vi "Edit papers.vi"(8 "Error In":errorcluster, 11 "INI refnum in":T1) -> (0 "Error Out":errorcluster, 3 "INI refnum Out":T1)   [LabVIEW 2015]
uses:
  <vilib>/Utility/config.llb/Config Data RefNum.ctl
  Edit papers state.ctl
  <vilib>/Utility/miscctls.llb/LVMenuShortCut.ctl
  <vilib>/Utility/config.llb/NI_LVConfig.lvlib
panel:
  in  "Clear table":bool
  in  "Exit":bool
  in  "Discared changes":bool
  in  "Save":bool
  in  "Table Control":string[][](table)
  # "Edit papers\n\nThe table below shows all the newspapers you've subscribed to along with their costs. A blank cost field indicates that the paper isn't delivered on that day. Edit the table values as required, and then click Save."
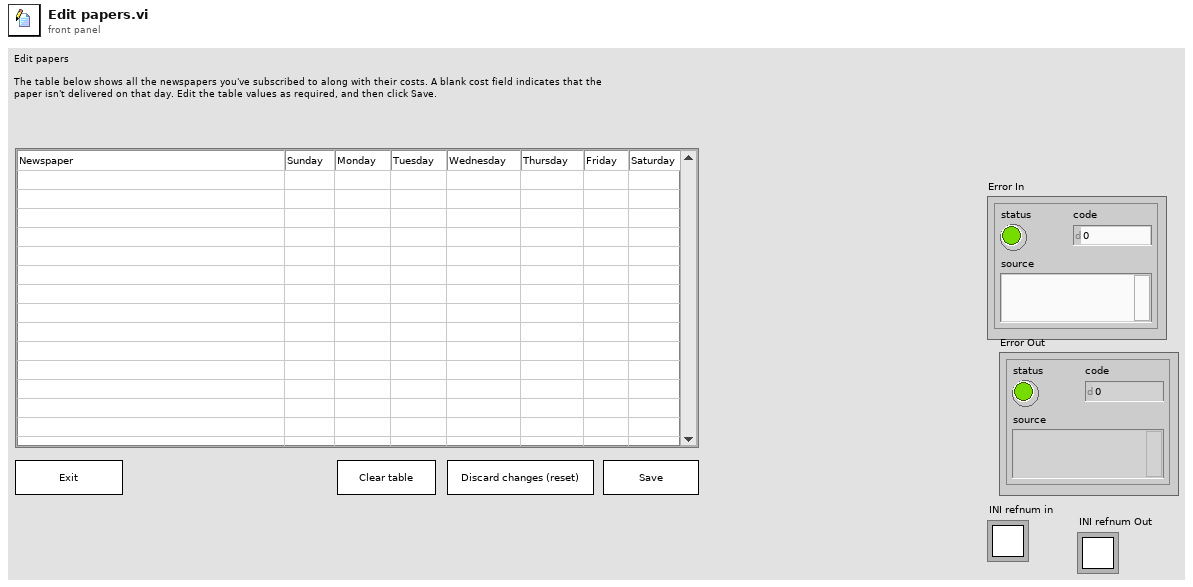
[diagram p1: front panel]
types:
  T1 = typedef "NI_LVConfig.lvlib/Config Data RefNum.ctl" = refnum<k1>
  T2 = typedef "Edit papers state.ctl" = enum16{"Init", "Idle", "Save", "Exit"}
  T3 = typedef "LVMenuShortCut.ctl" = cluster{"Include Shift Key?":bool, "Include Ctrl Key?":bool, "Shortcut Key":string}
  T4 = enum16{"Left Button", "Center Button", "Right Button", "Window Close"}
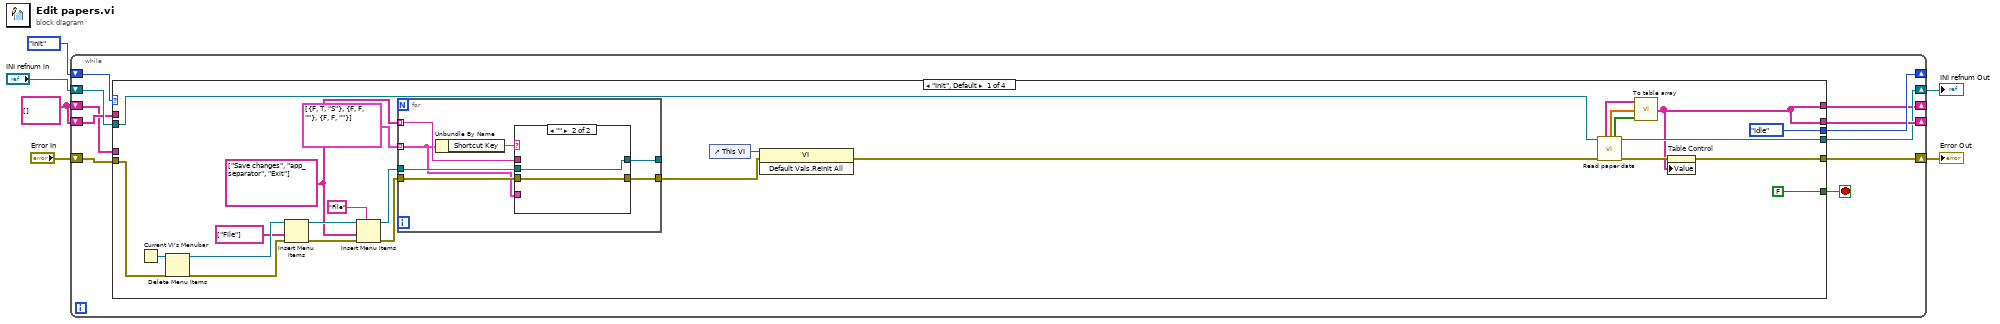
[diagram p0: block diagram]
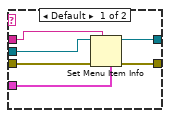
[diagram p2: hidden frame]
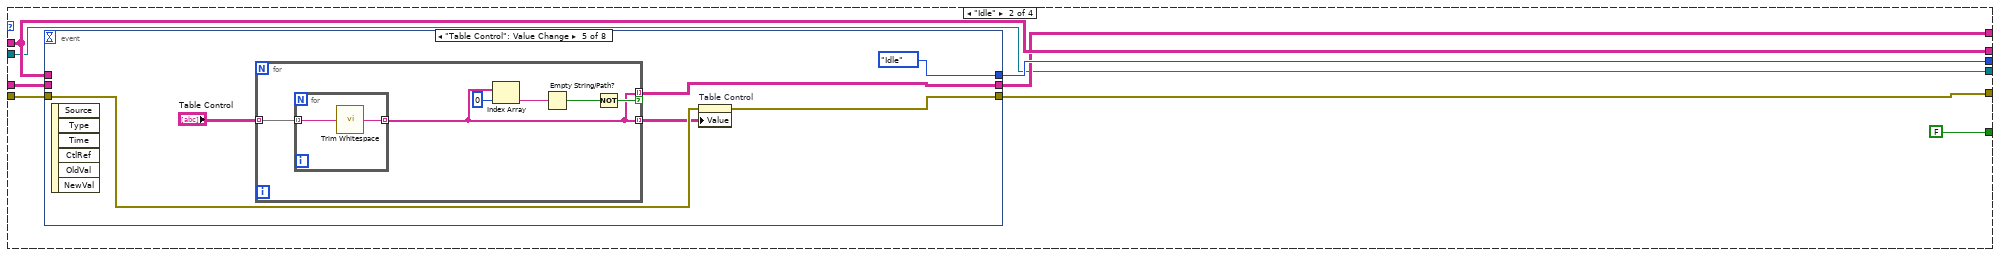
[diagram p3: hidden frame]
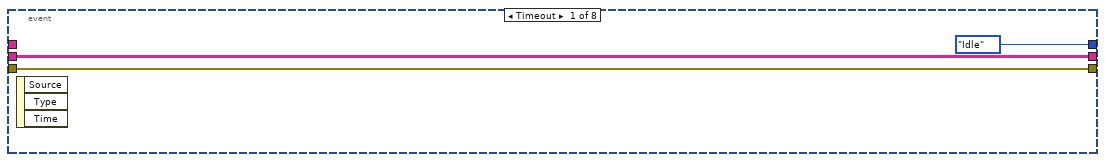
[diagram p4: hidden frame]
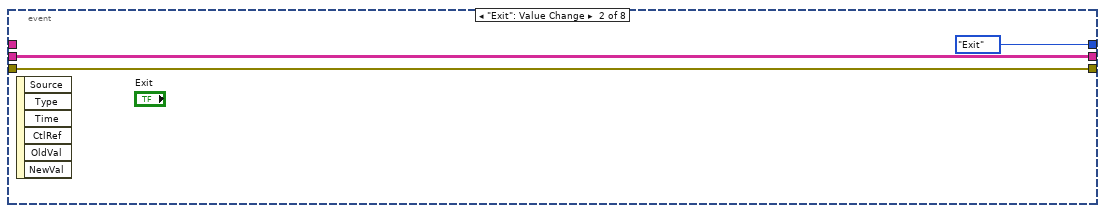
[diagram p5: hidden frame]
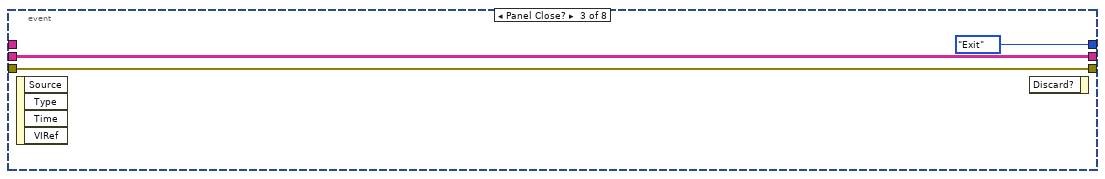
[diagram p6: hidden frame]
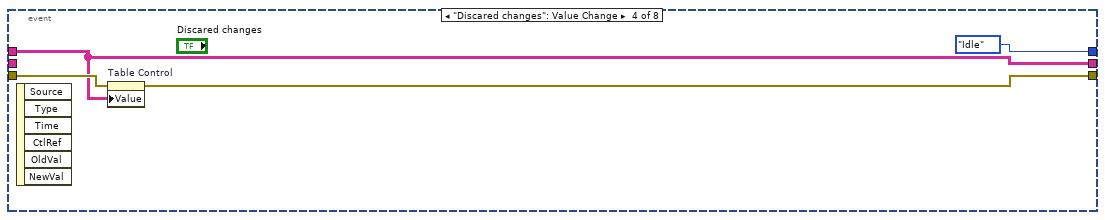
[diagram p7: hidden frame]
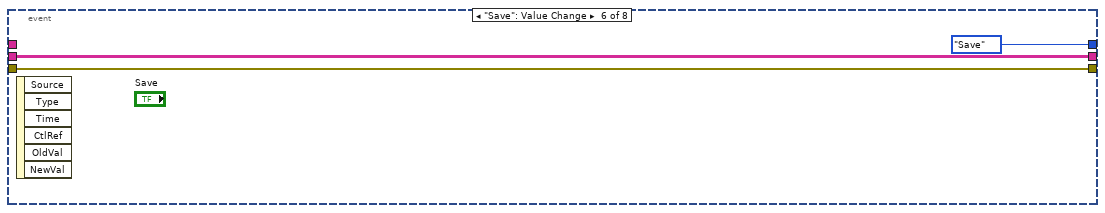
[diagram p8: hidden frame]
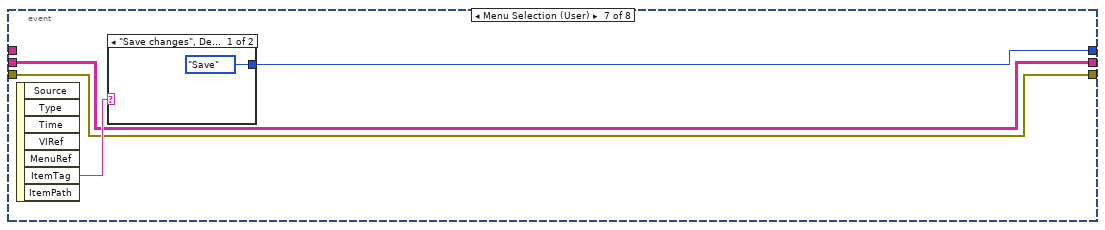
[diagram p9: hidden frame]
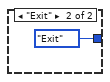
[diagram p10: hidden frame]
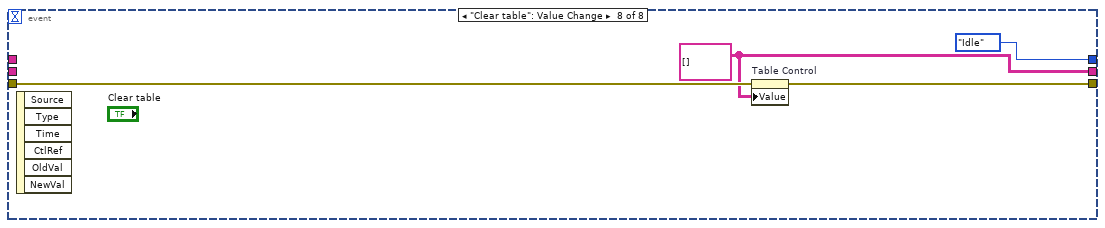
[diagram p11: hidden frame]
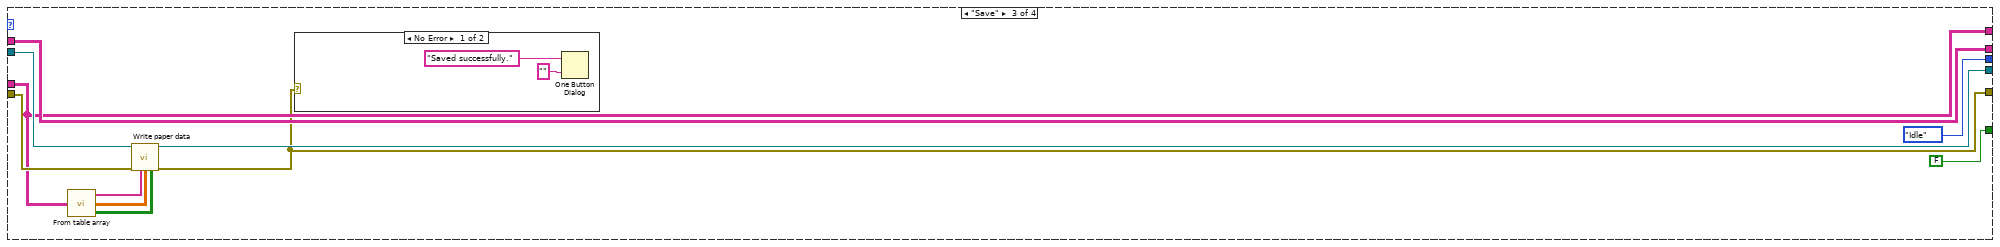
[diagram p12: hidden frame]
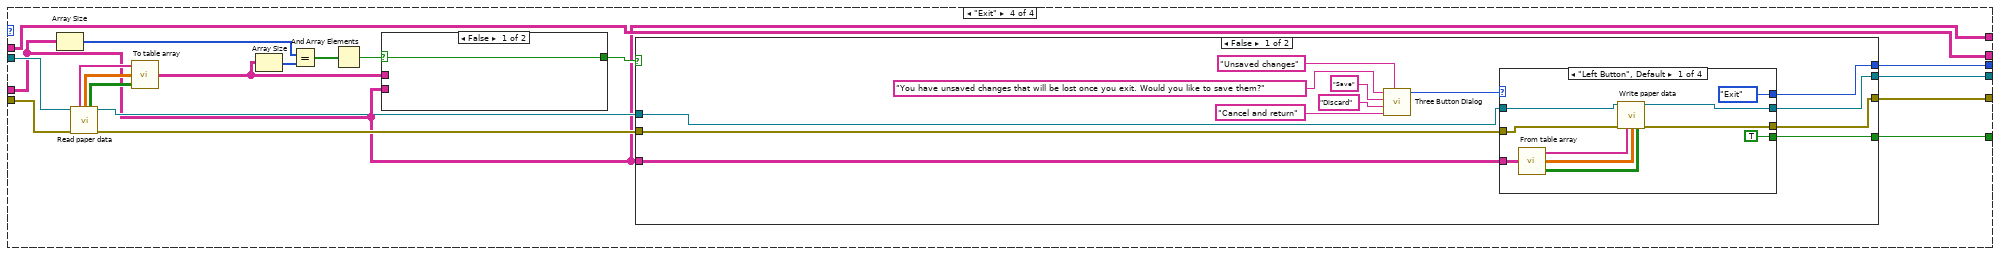
[diagram p14: hidden frame]
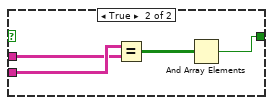
[diagram p15: hidden frame]
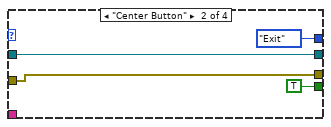
[diagram p16: hidden frame]
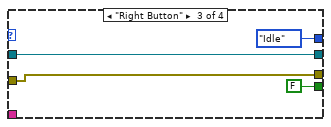
[diagram p17: hidden frame]
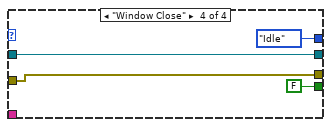
[diagram p18: hidden frame]
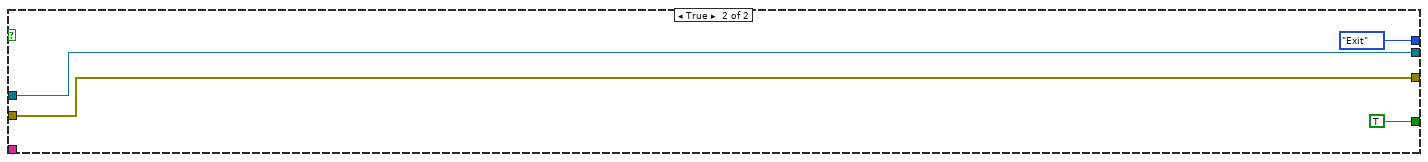
[diagram p19: hidden frame]
diagram:
  w3 = string[][] [] ("Table Array")
  n1 = while {
    shift-right: [w16] -> _
    shift-left: Edit_papers_state."Init" -> [w17]
    shift-right: [w11] -> w5
    shift-left: "Error In" -> [w14]
    shift-right: [w10] -> w4
    shift-left: "INI refnum in" -> [w15]
    shift-right: [w13] -> _
    shift-left: w3 -> [w12]
    shift-right: [w7] -> _
    shift-left: w3 -> [w9]
    stop <- w8 stop-if-true
    n2 = case shown="\"Init\", Default" w17 {
      tunnel: [Edit_papers_state."Idle" w65 Edit_papers_state."Idle" w134] -> w16
      tunnel: w15 -> [w40 w59 w114 w136]
      tunnel: w14 -> [w21 w63 w113 w135]
      tunnel: [w18 w64 w116 w137] -> w13
      tunnel: w12 -> [_ w64 w116 w137]
      tunnel: [w41 w62 w106 w130] -> w11
      tunnel: [w38 w59 w112 w129] -> w10
      tunnel: [w18 w61 w108 w120] -> w7
      tunnel: w9 -> [_ w60 w108 w120]
      tunnel: [FALSE FALSE FALSE w133] -> w8
      frame "Init", Default {
        w24 = string[] ["Save changes", "app_separator", "Exit"] ("item tags")
        n3 = Current VI's Menubar() -> (w33:refnum<k9>)
        n4 = Delete Menu Items(6:w21, 9:w33) -> (0:w32:errorcluster, 3:w31:refnum<k9>)  [unwired: 2 in]
        n5 = Insert Menu Items(6:w32, 7:string[] ["File"] ("item tags"), 9:w31) -> (0:w29:errorcluster, 3:w28:refnum<k9>)  [unwired: 3 in, 1 out]
        n6 = Insert Menu Items(5:"File" ("menu tag"), 6:w29, 7:w24, 9:w28) -> (0:w25:errorcluster, 3:w23:refnum<k9>)  [unwired: 2 in, 1 out]
        n7 = for {
          tunnel: w23 -> [w49]
          tunnel: w25 -> [w48]
          tunnel: w24 -> [w47] mode=indexing
          tunnel: T3[] [{"Include Shift Key?"=FALSE, "Include Ctrl Key?"=TRUE, "Shortcut Key"="S"}, {"Include Shift Key?"=FALSE, "Include Ctrl Key?"=FALSE, "Shortcut Key"=""}, {"Include Shift Key?"=FALSE, "Include Ctrl Key?"=FALSE, "Shortcut Key"=""}] ("short cut") -> [w44] mode=indexing
          tunnel: [w46] -> _
          tunnel: [w45] -> w22
          n8 = Unbundle By Name(w44) -> ("Shortcut Key"=w43:string)
          n9 = case shown="\"\"" w43 {
            tunnel: w49 -> [w55 w57]
            tunnel: w48 -> [w54 w56]
            tunnel: w47 -> [w53 _]
            tunnel: w44 -> [w52 _]
            tunnel: [w51 w57] -> w46
            tunnel: [w50 w56] -> w45
            frame Default {
              n10 = Set Menu Item Info(4:w52, 7:w53, 8:w54, 11:w55) -> (0:w50:errorcluster, 3:w51:refnum<k9>)  [unwired: 3 in]
            }
            frame "" {
            }
          }
        }
        n11 = control-ref of="This VI"() -> (w19:refnum<vi>)
        n12 = invoke class="VI" method="Default Vals.Reinit All"(reference=w19, error in=w22) -> (error out=w20:errorcluster)  [unwired: 1 in, 2 out]
        n13 = call "Read paper data.vi"("Refnum in"=w40, "error in (no error)"=w20) -> ("Names"=w37:string[], "Costs"=w36:dbl[][], "Days"=w35:bool[][], "Refnum out"=w38:T1, "error out"=w39:errorcluster)  [unwired: 9 in]
        n14 = call "To table array.vi"("Days"=w35, "Costs"=w36, "Names"=w37) -> ("Table Array"=w18:string[][])
        n15 = property on="Table Control" class="Tbl (strict)"(error in=w39, "Value"=w18) -> (error out=w41:errorcluster)  [unwired: 1 in, 1 out]
      }
      frame "Idle" {
        n16 = event shown="[4] \"Table Control\": Value Change" {
          selector: _ -> [_ _ _ _ _ _ _ _]
          dyn-events: _ -> [_ _ _ _ _ _ _ _]
          timeout: _ -> [_ _ _ _ _ _ _ _]
          tunnel: [Edit_papers_state."Idle" Edit_papers_state."Exit" Edit_papers_state."Exit" Edit_papers_state."Idle" Edit_papers_state."Idle" Edit_papers_state."Save" w96 Edit_papers_state."Idle"] -> w65
          tunnel: w64 -> [_ _ _ w75 _ _ _ _]
          tunnel: w63 -> [w66 w69 w72 w77 w82 w93 w97 w105]
          tunnel: [w66 w69 w72 w76 w81 w93 w97 w104] -> w62
          tunnel: [w67 w70 w73 w75 w83 w94 w98 w103] -> w61
          tunnel: w60 -> [w67 w70 w73 _ _ w94 w98 _]
          event Timeout {
            n17 = event-data() -> ()  [unwired: 1 in, 3 out]
          }
          event "Exit": Value Change {
            n18 = event-data() -> ()  [unwired: 1 in, 6 out]
          }
          event Panel Close? {
            n19 = event-data() -> ()  [unwired: 1 in, 4 out]
            n20 = event-data() -> ()  [unwired: 2 in, 1 out]
          }
          event "Discared changes": Value Change {
            n21 = event-data() -> ()  [unwired: 1 in, 6 out]
            n22 = property on="Table Control" class="Tbl (strict)"(error in=w77, "Value"=w75) -> (error out=w76:errorcluster)  [unwired: 1 in, 1 out]
          }
          event "Table Control": Value Change {
            n23 = event-data() -> ()  [unwired: 1 in, 6 out]
            n24 = for {
              tunnel: "Table Control" -> [w90] mode=indexing
              tunnel: [w85] -> w83 mode=indexing if=w87
              tunnel: [w85] -> w79 mode=indexing
              n25 = for {
                tunnel: w90 -> [w92] mode=indexing
                tunnel: [w91] -> w85 mode=indexing
                n26 = call <vilib>:"Trim Whitespace.vi"("string"=w92) -> ("trimmed string"=w91:string)  [unwired: 1 in]
              }
              n27 = Index Array(array=w85, index=0) -> (element=w89:string)
              n28 = Empty String/Path?(string/path=w89) -> (empty?=w88:bool)
              n29 = Not(x=w88) -> (.not. x?=w87:bool)
            }
            n30 = property on="Table Control" class="Tbl (strict)"(error in=w82, "Value"=w79) -> (error out=w81:errorcluster)  [unwired: 1 in, 1 out]
          }
          event "Save": Value Change {
            n31 = event-data() -> ()  [unwired: 1 in, 6 out]
          }
          event Menu Selection (User) {
            n32 = event-data() -> ("ItemTag"=w99:string)  [unwired: 1 in, 6 out]
            n33 = case shown="\"Save changes\", Default" w99 {
              tunnel: [Edit_papers_state."Save" Edit_papers_state."Exit"] -> w96
              frame "Save changes", Default {
              }
              frame "Exit" {
              }
            }
          }
          event "Clear table": Value Change {
            w103 = string[][] [] ("Table Array")
            n34 = event-data() -> ()  [unwired: 1 in, 6 out]
            n35 = property on="Table Control" class="Tbl (strict)"(error in=w105, "Value"=w103) -> (error out=w104:errorcluster)  [unwired: 1 in, 1 out]
          }
        }
      }
      frame "Save" {
        n36 = call "From table array.vi"("Table Array in"=w108) -> ("Names"=w111:string[], "Costs"=w110:dbl[][], "Days"=w109:bool[][])
        n37 = call "Write paper data.vi"("Refnum in"=w114, "error in (no error)"=w113, "Names"=w111, "Costs"=w110, "Days"=w109) -> ("Refnum out"=w112:T1, "error out"=w106:errorcluster)  [unwired: 9 in]
        n38 = case shown="No Error" w106 {
          frame No Error {
            n39 = One Button Dialog(message="Saved successfully.", button name ("OK")="") -> ()  [unwired: 1 out]
          }
          frame Error {
          }
        }
      }
      frame "Exit" {
        n40 = Array Size(array=w120) -> (size(s)=w124:i32[])
        n41 = call "Read paper data.vi"("Refnum in"=w136, "error in (no error)"=w135) -> ("Names"=w128:string[], "Costs"=w127:dbl[][], "Days"=w126:bool[][], "Refnum out"=w132:T1, "error out"=w131:errorcluster)  [unwired: 9 in]
        n42 = call "To table array.vi"("Days"=w126, "Costs"=w127, "Names"=w128) -> ("Table Array"=w119:string[][])
        n43 = Array Size(array=w119) -> (size(s)=w123:i32[])
        n44 = Equal?(x=w124, y=w123) -> (x = y?=w125:bool[])
        n45 = And Array Elements(Boolean array=w125) -> (logical AND=w122:bool)
        n46 = case shown="False" w122 {
          selector: w122 -> [w138 _]
          tunnel: [w138 w142] -> w121
          tunnel: w120 -> [_ w140]
          tunnel: w119 -> [_ w139]
          frame False {
          }
          frame True {
            n47 = Equal?(x=w140, y=w139) -> (x = y?=w141:bool[][])
            n48 = And Array Elements(Boolean array=w141) -> (logical AND=w142:bool)
          }
        }
        n49 = case shown="False" w121 {
          tunnel: [w144 Edit_papers_state."Exit"] -> w134
          tunnel: [w143 TRUE] -> w133
          tunnel: w120 -> [w149 _]
          tunnel: w132 -> [w148 w179]
          tunnel: w131 -> [w147 w178]
          tunnel: [w146 w178] -> w130
          tunnel: [w145 w179] -> w129
          frame False {
            n50 = call <vilib>:"Three Button Dialog.vi"("Window Title (\"\")"="Unsaved changes" ("Window Title (\"\")"), "Right Button Text (\"Cancel\")"="Cancel and return" ("Right Button Text (\"Cancel\")"), "Center Button Text (\"No\")"="Discard" ("Center Button Text (\"No\")"), "Left Button Text (\"Yes\")"="Save" ("Left Button Text (\"Yes\")"), "message"="You have unsaved changes that will be lost once you exit. Would you like to save them?") -> ("Which Button?"=w150:T4)  [unwired: 6 in]
            n51 = case shown="\"Left Button\", Default" w150 {
              tunnel: w149 -> [w165 _ _ _]
              tunnel: w148 -> [w161 w169 w173 w177]
              tunnel: w147 -> [w160 w168 w172 w176]
              tunnel: [w159 w168 w172 w176] -> w146
              tunnel: [w158 w169 w173 w177] -> w145
              tunnel: [Edit_papers_state."Exit" Edit_papers_state."Exit" Edit_papers_state."Idle" Edit_papers_state."Idle"] -> w144
              tunnel: [TRUE TRUE FALSE FALSE] -> w143
              frame "Left Button", Default {
                n52 = call "From table array.vi"("Table Array in"=w165) -> ("Names"=w164:string[], "Costs"=w163:dbl[][], "Days"=w162:bool[][])
                n53 = call "Write paper data.vi"("Refnum in"=w161, "error in (no error)"=w160, "Names"=w164, "Costs"=w163, "Days"=w162) -> ("Refnum out"=w158:T1, "error out"=w159:errorcluster)  [unwired: 9 in]
              }
              frame "Center Button" {
              }
              frame "Right Button" {
              }
              frame "Window Close" {
              }
            }
          }
          frame True {
          }
        }
      }
    }
  }
  "Error Out" <- w5
  "INI refnum Out" <- w4
